vi "8.LineMove.vi"() -> ()   [LabVIEW 2017]
uses:
  <vilib>/Platform/TimedLoop/XDataNode/timing_clust.ctl
  <vilib>/Platform/TimedLoop/XDataNode/nitl_modes.ctl
  <vilib>/Platform/TimedLoop/XDataNode/wakeup.ctl
  <vilib>/addons/control/pid/pid.llb/PID (DBL).vi
  <vilib>/Platform/TimedLoop/XDataNode/XDataNode.xnode
  <vilib>/Platform/TimedLoop/XDataNode/XDNodeRunTimeDep.lvlib
  <vilib>/ptbypt/NI_PtbyPt.lvlib
  <vilib>/addons/control/pid/NI_PID_pid.lvlib
panel:
  out "output":dbl caption="输出" format="%.2f"
  out "Y轴速度":dbl
  in  "停止":bool
  out "当前运行的距离":dbl(graph)
  in  "小车期望运\n行的距离":dbl caption="小车期望运行的距离" format="%.2f"
  in  "PID参数设定":T1={"proportional gain (Kc)"=8.0, "integral time (Ti, min)"=0.001, "derivative time (Td, min)"=0.0} caption="PID增益" {"derivative time (Td, min)" format="%.3f"; "integral time (Ti, min)" format="%.3f"; "proportional gain (Kc)" format="%.3f"}
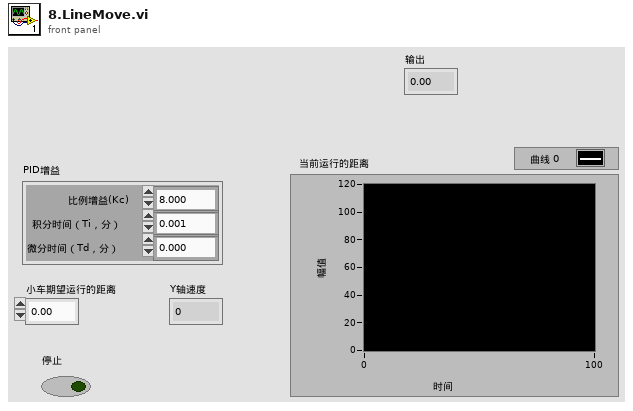
[diagram p1: front panel]
types:
  T1 = cluster{"proportional gain (Kc)":dbl, "integral time (Ti, min)":dbl, "derivative time (Td, min)":dbl}
  T2 = typedef "XDNodeRunTimeDep.lvlib/timing_clust.ctl" = cluster{"Expected End [f-1]":u64, "Actual End [f-1]":u64, "Finished Late? [f-1]":bool, "Expected End [i-1]":u64, "Actual End [i-1]":u64, "Finished Late? [i-1]":bool, "Expected Start [i]":u64, "Actual Start [i]":u64, "Expected Start [f]":u64, "Actual Start [f]":u64, "Source Name":string, "Structure Name":string, "Period":i64, "Deadline":i64, "Offset":i64, "Start":i64, "Priority":i32, "Timeout":i32, "Mode":T3, "Wakeup Reason":T4, "Error":errorcluster, "Source Type":string, "Secondary Source Type":string, "Global End Time":u64, "Global Start Time":u64, "Frame Duration":u64, "Iteration Duration":u64, "Assigned CPU":i32, "I/O Scan Engine Mode":u32}
  T3 = typedef "XDNodeRunTimeDep.lvlib/nitl_modes.ctl" = enum32{"No Change", "Process missed periods, maintain original phase", "Discard missed periods, maintain original phase", "Process missed periods, ignore original phase", "Discard missed periods, ignore original phase"}
  T4 = typedef "XDNodeRunTimeDep.lvlib/wakeup.ctl" = enum32{"Normal", "Aborted", "Asynchronous wakeup", "Timing source error", "Timed loop error", "Timeout"}
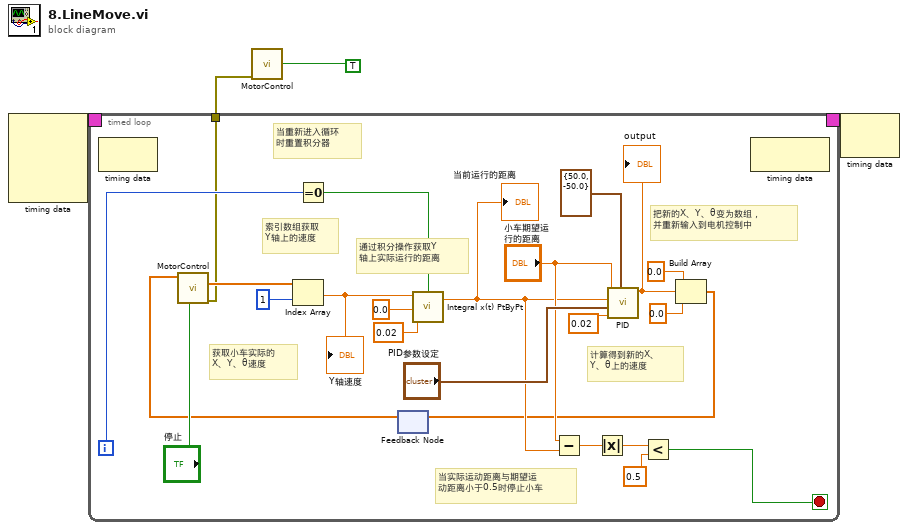
[diagram p0: block diagram]
diagram:
  n1 = node-c288() -> (w4:T2)  [unwired: 4 in]
  n2 = timed-loop {
    timing: w4 -> [_]
    timing-out: [_] -> w3
    tunnel: [w6] -> w1
    i -> [w15]
    stop <- w7 stop-if-true
    # "当实际运动距离与期望运\n动距离小于0.5时停止小车"
    # "把新的X、Y、θ变为数组，\n并重新输入到电机控制中"
    # "计算得到新的X、\nY、θ上的速度"
    # "当重新进入循环\n时重置积分器"
    # "通过积分操作获取Y\n轴上实际运行的距离"
    # "索引数组获取\nY轴上的速度"
    # "获取小车实际的\nX、Y、θ速度"
    n3 = node-c288() -> ()  [unwired: 1 in, 1 out]
    n4 = Equal To 0?(x=w15) -> (x = 0?=w22:bool)
    n5 = feedback #1() -> (w13:dbl[])  [unwired: 1 in]
    n6 = call "MotorControl.vi"("停止"="停止", "把当前坐标系下期望小\n车在X、Y、θ的速度作\n为逆运算的输入"=w13) -> ("error out"=w6:errorcluster, "真实坐标系下的X、Y、θ的速度"=w27:dbl[])  [unwired: 8 in]
    n7 = Index Array(array=w27, index=1 ("索引")) -> (element=w25:dbl)
    "Y轴速度" <- w25
    n8 = call <vilib>:"Integral x(t) PtByPt.vi"("initialize"=w22, "dt"=0.02, "initial condition"=0.0, "x"=w25) -> ("integral x(t)"=w11:dbl)  [unwired: 1 out]
    "当前运行的距离" <- w11
    n9 = Subtract(x="小车期望运\n行的距离", y=w11) -> (x-y=w10:dbl)
    n10 = Absolute Value(x=w10) -> (abs(x)=w9:dbl)
    n11 = call-poly <vilib>:"PID.vi"("output range"=cluster{"output high":dbl, "output low":dbl} {"output high"=50.0, "output low"=-50.0}, "dt (s)"=0.02, "PID gains"="PID参数设定", "process variable"=w11, "setpoint"="小车期望运\n行的距离") -> ("output"=w18:dbl)  [unwired: 5 in, 1 out]
    "output" <- w18
    n12 = Less?(x=w9, y=0.5) -> (x < y?=w7:bool)
    n13 = Build Array(0.0 ("元素"), w18, 0.0 ("元素")) -> (w5:dbl[])
    n14 = feedback-in #1(w5) -> ()
    n15 = node-c288() -> ()  [unwired: 1 in, 1 out]
  }
  n16 = call "MotorControl.vi"("停止"=TRUE, "error in (no error)"=w1) -> ()  [unwired: 8 in, 2 out]
  n17 = node-c288(w3) -> ()  [unwired: 1 out]
